vi "Preset GR. CONT. test.vi"(8 "error in (no error)":errorcluster, 11 "VISA resource in":refnum<visa-resource-name>) -> (0 "error out":errorcluster, 3 "VISA resource out":refnum<visa-resource-name>)   [LabVIEW 2025]
doc: "This VI writes to the instrument the AC-V FREQ. value."
uses:
  <instrlib>/Chroma 19052/Chroma 19052.lvlib
panel:
  in  "Value":dbl min=0.0 max=99.9 step=0.1 format="%.1f"
  # "0=OFF\n0,1=KEY\n0,2-99,9 [s] time to START"
  # "Preset GROUND Resistance\nCONTINUITY query"
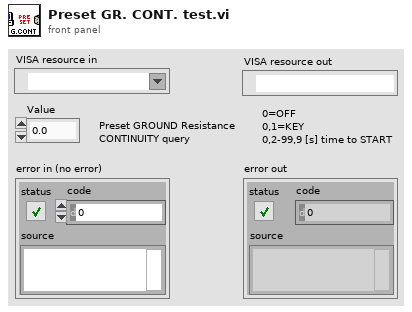
[diagram p1: front panel]
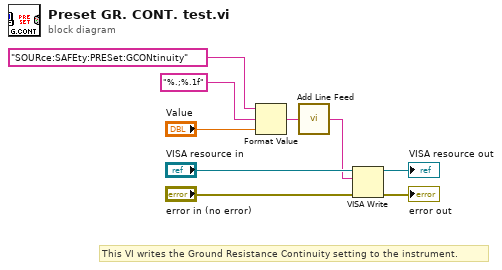
[diagram p0: block diagram]
diagram:
  # "This VI writes the Ground Resistance Continuity setting to the instrument."
  n1 = Format Value(string ("")="SOURce:SAFEty:PRESet:GCONtinuity", format string="%.;%.1f", value (0)="Value") -> (output string=w4:string)
  n2 = call <instrlib>:"Add Line Feed.vi"("Command string"=w4) -> ("Concatenated string"=w7:string)  [unwired: 4 in]
  n3 = VISA Write(VISA resource name="VISA resource in", write buffer=w7, error in (no error)="error in (no error)") -> (VISA resource name out=→"VISA resource out":refnum<visa-resource-name>, error out=→"error out":errorcluster)  [unwired: 1 out]
